vi "动态调用非模式对话框.vi"() -> ()   [LabVIEW 2013]
panel:
  out "错误输出":errorcluster
  in  "停止":bool
  out "波形图表":dbl(graph)
  in  "调用非模式对话框":bool
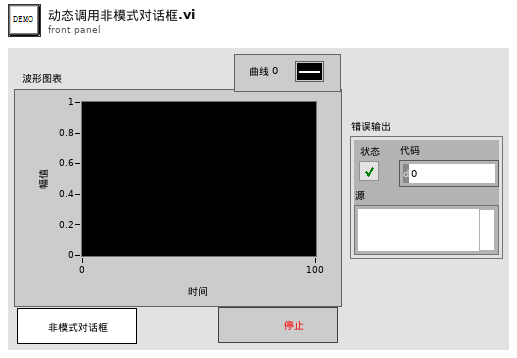
[diagram p1: front panel]
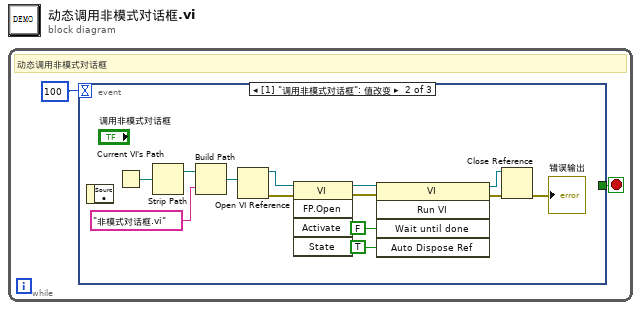
[diagram p0: block diagram]
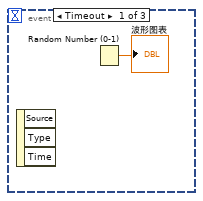
[diagram p2: hidden frame]
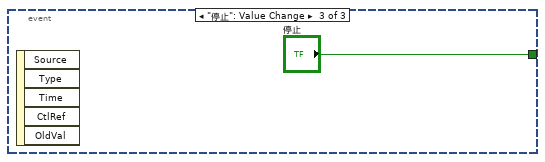
[diagram p3: hidden frame]
diagram:
  n1 = while {
    stop <- w2 stop-if-true
    # "动态调用非模式对话框"
    n2 = event shown="[1] \"调用非模式对话框\": 值改变" {
      selector: _ -> [_ _ _]
      dyn-events: _ -> [_ _ _]
      timeout: 100 -> [_ _ _]
      tunnel: [_ _ "停止"] -> w2
      event Timeout {
        n3 = event-data() -> ()  [unwired: 1 in, 3 out]
        n4 = Random Number (0-1)() -> (number: 0 to 1=→"波形图表":dbl)
      }
      event "调用非模式对话框": Value Change {
        n5 = event-data() -> ()  [unwired: 1 in, 1 out]
        n6 = Current VI's Path() -> (path=w16:path)
        n7 = Strip Path(path=w16) -> (stripped path=w15:path)  [unwired: 1 out]
        n8 = Build Path(base path=w15, name or relative path="非模式对话框.vi" ("名称或相对路径")) -> (appended path=w13:path)
        n9 = Open VI Reference(vi path=w13) -> (vi reference=w7:refnum<vi>, error out=w6:errorcluster)  [unwired: 5 in]
        n10 = invoke class="VI" method="FP.Open"(reference=w7, error in=w6) -> (reference out=w5:refnum<vi>, error out=w4:errorcluster)  [unwired: 3 in, 3 out]
        n11 = invoke class="VI" method="Run VI"(reference=w5, error in=w4, "Wait until done"=FALSE ("结束前等待"), "Auto Dispose Ref"=TRUE ("自动销毁引用")) -> (reference out=w9:refnum<vi>, error out=w10:errorcluster)  [unwired: 1 in, 3 out]
        n12 = Close Reference(reference=w9, error in (no error)=w10) -> (error out=→"错误输出":errorcluster)
      }
      event "停止": Value Change {
        n13 = event-data() -> ()  [unwired: 1 in, 5 out]
      }
    }
  }
